vi "Autonomous - Get Mode.vi"(0 "Autonomous Selector Value":u8) -> (1 "Autonomous Mode":T1)   [LabVIEW 2015]
uses:
  Autonomous Mode.ctl
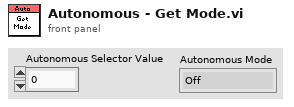
[diagram p1: front panel]
types:
  T1 = typedef "Autonomous Mode.ctl" = enum16{"Off", "Cross Defense", "Shoot A/B", "Shoot C/D", "Shoot E"}
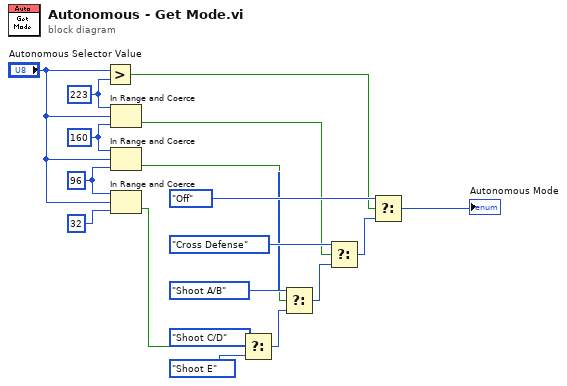
[diagram p0: block diagram]
diagram:
  w5 = u8 223 ("upper limit")
  w4 = u8 160 ("upper limit")
  w3 = u8 96 ("upper limit")
  n1 = Greater?(x="Autonomous Selector Value", y=w5) -> (0:w14:bool)
  n2 = In Range and Coerce(upper limit=w5, x="Autonomous Selector Value", lower limit=w4) -> (In Range?=w13:bool)  [unwired: 1 out]
  n3 = In Range and Coerce(upper limit=w4, x="Autonomous Selector Value", lower limit=w3) -> (In Range?=w12:bool)  [unwired: 1 out]
  n4 = In Range and Coerce(upper limit=w3, x="Autonomous Selector Value", lower limit=u8 32 ("upper limit")) -> (In Range?=w8:bool)  [unwired: 1 out]
  n5 = Select(t=Autonomous_Mode."Shoot C/D", s=w8, f=Autonomous_Mode."Shoot E") -> (s? t:f=w9:T1)
  n6 = Select(t=Autonomous_Mode."Shoot A/B", s=w12, f=w9) -> (s? t:f=w10:T1)
  n7 = Select(t=Autonomous_Mode."Cross Defense", s=w13, f=w10) -> (s? t:f=w11:T1)
  n8 = Select(t=Autonomous_Mode."Off", s=w14, f=w11) -> (s? t:f=→"Autonomous Mode":T1)
